vi "OTG Reader.vi"(8 "error in (no error)":errorcluster, 11 "OTG File Path":path=path "" caption="start path") -> (0 "Read Spreadsheet Error":errorcluster, 3 "Opto 22 Rack Array":T1(array[cluster]))   [LabVIEW 2024, in "OptoMMP.lvlib"]
doc: "Takes a file path to a PAC Manager OTG file and returns an array of clusters each containing an IP address for the Opto 22 rack controller, an array of channel types (AIN/AOUT, DIN/DOUT, etc.) and an array of rack point numbers corresponding to the channel types.\n\nLast updated: 7/25/2025"
uses:
  <instrlib>/OptoMMP/OptoMMP.lvlib
  <vilib>/Utility/file.llb/Read Delimited Spreadsheet (string).vi
panel:
  # "Copyright (c) 2025 California Institute of Technology (Caltech).\nU.S. Government sponsorship acknowledged.\n\nLicensed under the Apache License, Version 2.0 (the \"License\");\nyou may not use this file except in compliance with the License.\nYou may obtain a copy of the License at\n\n    http://www.apache.org/licenses/LICENSE-2.0\n\nUnless required by applicable law or agreed to in writing, software\ndistributed under the License is distributed on an \"AS IS\" BASIS,\nWITHOUT WARRANTIES OR CONDITIONS OF ANY KIND, either express or implied.\nSee the License for the specific language governing permissions and\nlimitations under the License."
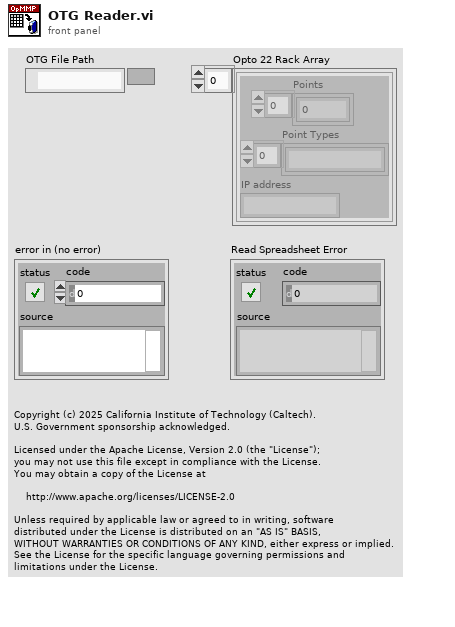
[diagram p1: front panel]
types:
  T1 = cluster{"Points":i32[], "Point Types":string[], "IP address":string}[]
  T2 = cluster{"Points":i32[], "Point Types":string[], "IP Addresses":string}
  T3 = cluster{"Points":i32[], "Point Types":string[], "IP Addresses":string}[]
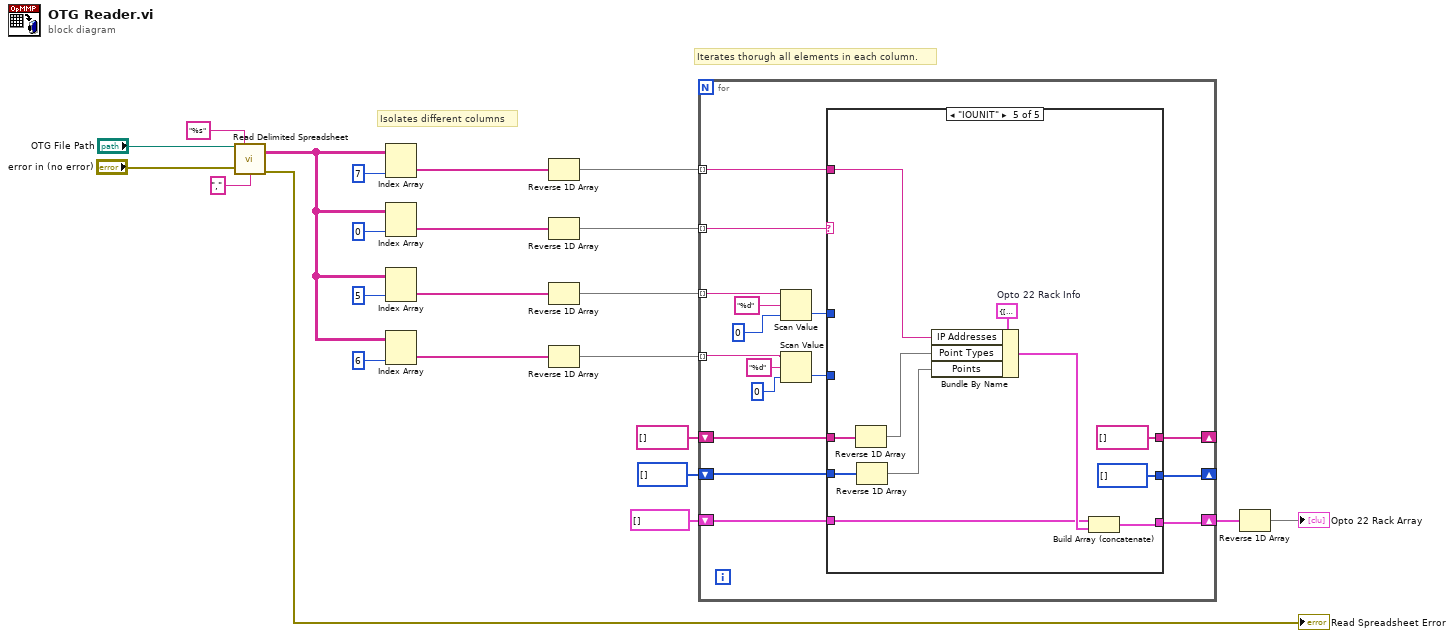
[diagram p0: block diagram]
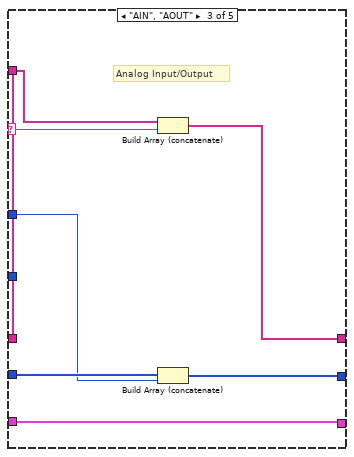
[diagram p4: hidden frame]
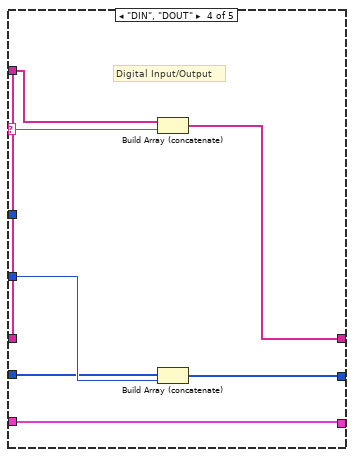
[diagram p5: hidden frame]
diagram:
  # "Isolates different columns"
  # "Iterates thorugh all elements in each column."
  n1 = call-poly <vilib>:"Read Delimited Spreadsheet.vi"("file path (dialog if empty)"="OTG File Path", "format (%s)"="%s", "error in (no error)"="error in (no error)", "delimiter (\\t)"="," ("delimiter (\\t)")) -> ("all rows"=w4:string[][], "error out"=→"Read Spreadsheet Error":errorcluster)  [unwired: 6 in, 4 out]
  n2 = Index Array(array=w4, index (col)=7 ("index")) -> (element=w7:string[])  [unwired: 1 in]
  n3 = Index Array(array=w4, index (col)=0 ("index")) -> (element=w8:string[])  [unwired: 1 in]
  n4 = Index Array(array=w4, index (col)=5 ("index")) -> (element=w12:string[])  [unwired: 1 in]
  n5 = Index Array(array=w4, index (col)=6 ("index")) -> (element=w14:string[])  [unwired: 1 in]
  n6 = Reverse 1D Array(array=w7) -> (reversed array=w18:string[])
  n7 = Reverse 1D Array(array=w8) -> (reversed array=w15:string[])
  n8 = Reverse 1D Array(array=w12) -> (reversed array=w16:string[])
  n9 = Reverse 1D Array(array=w14) -> (reversed array=w17:string[])
  n10 = for {
    tunnel: w15 -> [w39] mode=indexing
    tunnel: w18 -> [w38] mode=indexing
    tunnel: w16 -> [w35] mode=indexing
    tunnel: w17 -> [w29] mode=indexing
    shift-right: [w37] -> _
    shift-left: i32[] [] -> [w36]
    shift-right: [w26] -> w20
    shift-left: T1 [] -> [w27]
    shift-right: [w25] -> _
    shift-left: string[] [] -> [w24]
    n11 = Scan Value(string=w35, format string="%d", default (0 dbl)=0) -> (value=w32:i32)  [unwired: 1 out]
    n12 = Scan Value(string=w29, format string="%d", default (0 dbl)=0) -> (value=w28:i32)  [unwired: 1 out]
    n13 = case shown="\"IOUNIT\"" w39 {
      selector: w39 -> [_ _ w46 w54 _]
      tunnel: w38 -> [_ _ _ _ w62]
      tunnel: w32 -> [_ _ w47 _ _]
      tunnel: w28 -> [_ _ _ w59 _]
      tunnel: [w42 w45 w49 w58 i32[] []] -> w37
      tunnel: w36 -> [w42 w45 w48 w57 w64]
      tunnel: w27 -> [w41 w44 w52 w56 w68]
      tunnel: [w41 w44 w52 w56 w67] -> w26
      tunnel: [w40 w43 w50 w55 string[] []] -> w25
      tunnel: w24 -> [w40 w43 w51 w53 w65]
      frame Default {
      }
      frame "DEVICECONNECTION" {
      }
      frame "AIN", "AOUT" {
        # "Analog Input/Output"
        n14 = Build Array (concatenate)(w51, w46) -> (w50:string[])
        n15 = Build Array (concatenate)(w48, w47) -> (w49:i32[])
      }
      frame "DIN", "DOUT" {
        # "Digital Input/Output"
        n16 = Build Array (concatenate)(w53, w54) -> (w55:string[])
        n17 = Build Array (concatenate)(w57, w59) -> (w58:i32[])
      }
      frame "IOUNIT" {
        w66 = T2 {"Points"=[], "Point Types"=[], "IP Addresses"=""}  # Opto 22 Rack Info
        n18 = Reverse 1D Array(array=w65) -> (reversed array=w60:string[])
        n19 = Reverse 1D Array(array=w64) -> (reversed array=w61:i32[])
        n20 = Bundle By Name(cluster=w66, "IP Addresses"=w62, "Point Types"=w60, "Points"=w61) -> (w69:T2)
        n21 = Build Array (concatenate)(w68, w69) -> (w67:T3)
      }
    }
  }
  n22 = Reverse 1D Array(array=w20) -> (reversed array=→"Opto 22 Rack Array":T1)
